vi "ws_parse user credentials.vi"(7 "httpRequestID":u32, 8 "error in (no error)":errorcluster, 9 "Force Logout? (f)":bool, 11 "DB Connection Ref":T1) -> (0 "error out":errorcluster, 1 "Login?":bool, 3 "dup DB Connection Ref":T1, 4 "User":T2)   [LabVIEW 2011]
uses:
  server/database/Users/User Record.ctl
  SI.LIB/ODBC/SQL Controls/Connection Refnum.ctl
  <vilib>/wsapi/subVIs/Write Single Session Variable.vi
  <vilib>/wsapi/NI_WebServices.lvlib
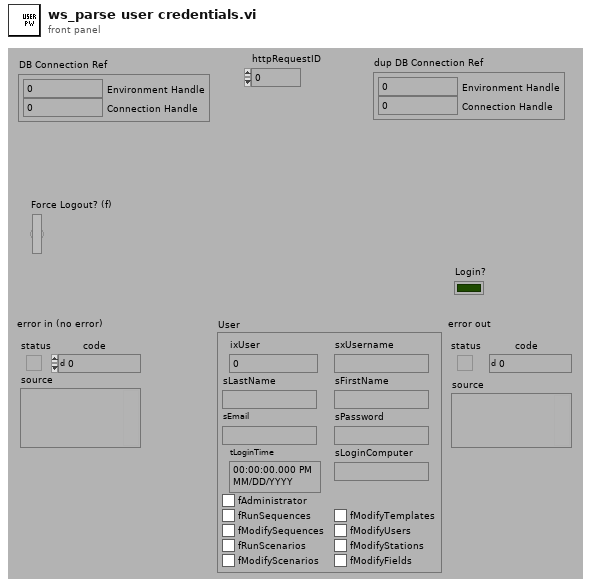
[diagram p1: front panel]
types:
  T1 = typedef "Connection Refnum.ctl" = cluster{"Environment Handle":i32, "Connection Handle":i32}
  T2 = typedef "User Record.ctl" = cluster{"ixUser":i32, "sxUsername":string, "sLastName":string, "sFirstName":string, "sEmail":string, "sPassword":string, "tLoginTime":timestamp, "sLoginComputer":string, "fAdministrator":bool, "fRunSequences":bool, "fModifySequences":bool, "fRunScenarios":bool, "fModifyScenarios":bool, "fModifyTemplates":bool, "fModifyUsers":bool, "fModifyStations":bool, "fModifyFields":bool}
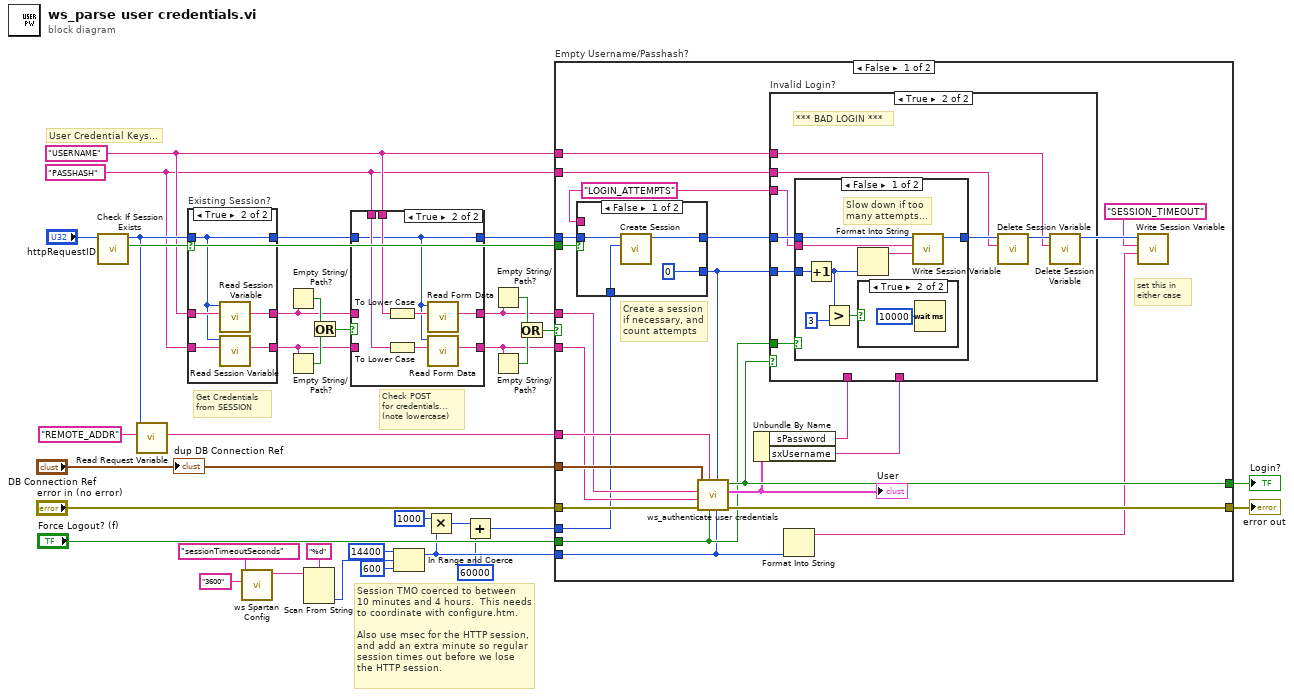
[diagram p0: block diagram]
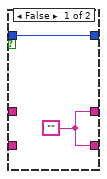
[diagram p3: hidden frame]
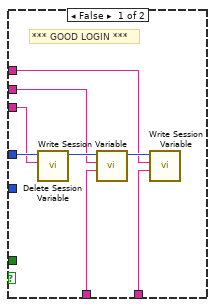
[diagram p4: hidden frame]
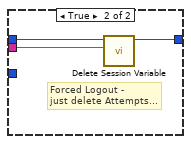
[diagram p6: hidden frame]
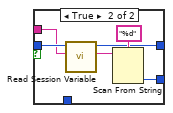
[diagram p7: hidden frame]
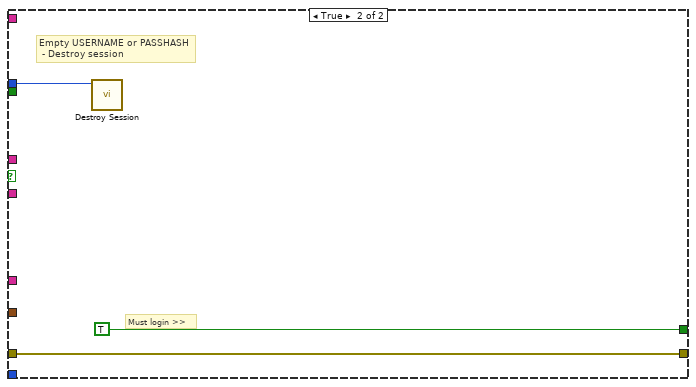
[diagram p8: hidden frame]
diagram:
  w19 = "PASSHASH"
  w20 = "USERNAME"
  # "Session TMO coerced to between\n10 minutes and 4 hours.  This needs\nto coordinate with configure.htm.\n\nAlso use msec for the HTTP session, \nand add an extra minute so regular\nsession times out before we lose\nthe HTTP session."
  # "Get Credentials\nfrom SESSION"
  # "Check POST\nfor credentials...\n(note lowercase)"
  # "User Credential Keys..."
  n1 = call <vilib>:"Check If Session Exists.vi"("httpRequestID"="httpRequestID") -> ("session exists?"=w23:bool, "httpRequestID out"=w22:u32)  [unwired: 8 in, 1 out]
  n2 = call <vilib>:"Read Request Variable.vi"("variable name"="REMOTE_ADDR" ("Spartan User Credential Cookie"), "httpRequestID"=w22) -> ("value"=w29:string)  [unwired: 7 in, 2 out]
  n3 = case "Existing Session?" shown="True" w23 {
    tunnel: w22 -> [w38 w41]
    tunnel: [w38 w41] -> w21
    tunnel: w20 -> [_ w43]
    tunnel: w19 -> [_ w42]
    tunnel: [w37 w40] -> w16
    tunnel: [w37 w39] -> w15
    frame False {
      w37 = ""
    }
    frame True {
      n4 = call <vilib>:"Read Session Variable.vi"("key"=w43, "httpRequestID"=w41) -> ("value"=w40:string)  [unwired: 7 in, 2 out]
      n5 = call <vilib>:"Read Session Variable.vi"("key"=w42, "httpRequestID"=w41) -> ("value"=w39:string)  [unwired: 7 in, 2 out]
    }
  }
  n6 = call "ws Spartan Config.vi"("default value (\"\")"="3600" ("default value"), "config key (\"\")"="sessionTimeoutSeconds") -> ("config value"=w10:string)  [unwired: 7 in, 2 out]
  n7 = Empty String/Path?(string/path=w16) -> (empty?=w18:bool)
  n8 = Empty String/Path?(string/path=w15) -> (empty?=w17:bool)
  n9 = Scan From String(format string="%d", input string=w10) -> (output 1=w8:i32)  [unwired: 2 in, 4 out]
  n10 = Or(x=w18, y=w17) -> (x .or. y?=w14:bool)
  n11 = case shown="True" w14 {
    tunnel: [w46 w53] -> w31
    tunnel: [w45 w52] -> w30
    tunnel: w21 -> [w44 w47]
    tunnel: w20 -> [_ w49]
    tunnel: w19 -> [_ w48]
    tunnel: w16 -> [w46 _]
    tunnel: w15 -> [w45 _]
    tunnel: [w44 w47] -> w13
    frame False {
      # "Existing session\ncred's override\nPOSTed cred's"
    }
    frame True {
      n12 = To Lower Case(string=w49) -> (all lower case string=w50:string)
      n13 = To Lower Case(string=w48) -> (all lower case string=w51:string)
      n14 = call <vilib>:"Read Form Data.vi"("key"=w50, "httpRequestID"=w47) -> ("value"=w53:string)  [unwired: 7 in, 2 out]
      n15 = call <vilib>:"Read Form Data.vi"("key"=w51, "httpRequestID"=w47) -> ("value"=w52:string)  [unwired: 7 in, 2 out]
    }
  }
  n16 = In Range and Coerce(upper limit=14400, x=w8, lower limit=600) -> (coerced(x)=w5:i32)  [unwired: 1 out]
  n17 = Multiply(x=1000, y=w5) -> (x*y=w2:i32)
  n18 = Add(x=w2, y=60000 ("lower limit")) -> (x+y=w3:i32)
  n19 = Empty String/Path?(string/path=w31) -> (empty?=w35:bool)
  n20 = Empty String/Path?(string/path=w30) -> (empty?=w34:bool)
  n21 = Or(x=w35, y=w34) -> (x .or. y?=w32:bool)
  n22 = case "Empty Username/Passhash?" shown="False" w32 {
    tunnel: w13 -> [w75 w116]
    tunnel: w31 -> [w64 _]
    tunnel: w30 -> [w63 _]
    tunnel: w23 -> [w74 _]
    tunnel: w20 -> [w73 _]
    tunnel: w19 -> [w72 _]
    tunnel: w29 -> [w65 _]
    tunnel: "error in (no error)" -> [w70 w114]
    tunnel: [w69 w114] -> w28
    tunnel: [w68 TRUE] -> w27
    tunnel: "DB Connection Ref" -> [w67 _]
    tunnel: "Force Logout? (f)" -> [w59 _]
    tunnel: w5 -> [w58 _]
    tunnel: w3 -> [w57 _]
    frame False {
      w71 = "LOGIN_ATTEMPTS"
      # "set this in\neither case"
      # "Create a session\nif necessary, and\ncount attempts"
      n23 = case shown="False" w74 {
        tunnel: w75 -> [w107 w111]
        tunnel: [w106 w110] -> w56
        tunnel: w71 -> [_ w109]
        tunnel: [0 ("output 1") w108] -> w66
        tunnel: w57 -> [w104 _]
        frame False {
          n24 = call <vilib>:"Create Session.vi"("timeout (60000 msec)"=w104, "httpRequestID"=w107) -> ("httpRequestID out"=w106:u32)  [unwired: 7 in, 2 out]
        }
        frame True {
          n25 = call <vilib>:"Read Session Variable.vi"("key"=w109, "httpRequestID"=w111) -> ("value"=w112:string, "httpRequestID out"=w110:u32)  [unwired: 7 in, 1 out]
          n26 = Scan From String(format string="%d", input string=w112) -> (output 1=w108:i32)  [unwired: 3 in, 3 out]
        }
      }
      n27 = call "ws_authenticate user credentials.vi"("Session Timeout, Seconds (0)"=w58, "Attempts (0)"=w66, "Force Logout? (f)"=w59, "REMOTE_ADDR (\"\")"=w65, "error in (no error)"=w70, "Passhash (\"\")"=w63, "Username (\"\")"=w64, "DB Connection Ref"=w67) -> ("error out"=w69:errorcluster, "User Record"=w62:T2, "User must login?"=w68:bool)  [unwired: 1 in]
      "User" <- w62
      n28 = Unbundle By Name(w62) -> ("sPassword"=w61:string, "sxUsername"=w60:string)
      n29 = case "Invalid Login?" shown="True" w68 {
        tunnel: w56 -> [w83 w90]
        tunnel: w71 -> [w82 w91]
        tunnel: w73 -> [w78 w86]
        tunnel: w72 -> [w79 w88]
        tunnel: w66 -> [_ w84]
        tunnel: w61 -> [w77 _]
        tunnel: w60 -> [w76 _]
        tunnel: w59 -> [_ w85]
        frame False {
          # "*** GOOD LOGIN ***"
          n30 = call <vilib>:"Delete Session Variable.vi"("key"=w82, "httpRequestID"=w83) -> ("httpRequestID out"=w80:u32)  [unwired: 8 in, 1 out]
          n31 = call-poly <vilib>:"Write Session Variable.vi"("value"=w77, "key"=w79, "httpRequestID"=w80) -> ("httpRequestID out"=w81:u32)  [unwired: 5 in, 3 out]
          n32 = call-poly <vilib>:"Write Session Variable.vi"("value"=w76, "key"=w78, "httpRequestID"=w81) -> ()  [unwired: 5 in, 4 out]
        }
        frame True {
          # "*** BAD LOGIN ***"
          n33 = case shown="False" w85 {
            tunnel: w91 -> [w99 w101]
            tunnel: w90 -> [w98 w103]
            tunnel: [w97 w102] -> w89
            tunnel: w84 -> [w94 _]
            frame False {
              # "Slow down if too\nmany attempts..."
              n34 = Increment(x=w94) -> (x+1=w93:i32)
              n35 = Greater?(x=w93, y=3) -> (0:w92:bool)
              n36 = Format Into String(w93) -> (resulting string=w96:string)  [unwired: 3 in, 1 out]
              n37 = case shown="True" w92 {
                frame False {
                }
                frame True {
                  n38 = Wait (ms)(milliseconds to wait=u32 10000) -> ()  [unwired: 1 out]
                }
              }
              n39 = call-poly <vilib>:"Write Session Variable.vi"("value"=w96, "key"=w99, "httpRequestID"=w98) -> ("httpRequestID out"=w97:u32)  [unwired: 5 in, 3 out]
            }
            frame True {
              # "Forced Logout -\njust delete Attempts..."
              n40 = call <vilib>:"Delete Session Variable.vi"("key"=w101, "httpRequestID"=w103) -> ("httpRequestID out"=w102:u32)  [unwired: 8 in, 1 out]
            }
          }
          n41 = call <vilib>:"Delete Session Variable.vi"("key"=w88, "httpRequestID"=w89) -> ("httpRequestID out"=w87:u32)  [unwired: 8 in, 1 out]
          n42 = call <vilib>:"Delete Session Variable.vi"("key"=w86, "httpRequestID"=w87) -> ()  [unwired: 8 in, 2 out]
        }
      }
      n43 = Format Into String(w58) -> (resulting string=w55:string)  [unwired: 3 in, 1 out]
      n44 = call-poly <vilib>:"Write Session Variable.vi"("value"=w55, "key"="SESSION_TIMEOUT", "httpRequestID"=w56) -> ()  [unwired: 5 in, 4 out]
    }
    frame True {
      # "Must login >>"
      # "Empty USERNAME or PASSHASH\n - Destroy session"
      n45 = call <vilib>:"Destroy Session.vi"("httpRequestID"=w116) -> ()  [unwired: 9 in, 2 out]
    }
  }
  "error out" <- w28
  "Login?" <- w27
  "dup DB Connection Ref" <- "DB Connection Ref"
